vi "CS_cRIO-PB_MSAC2_DPV1-InitiateReq.vi"(0 "FPGA VI Reference":T6, 5 "Slave":i8, 7 "Initiate data":T7={"Communication ref.:"=0, "Send timeout (x10ms):"=0, "Feat. supp. 1:"=0, "Feat. supp. 2:"=0, "Profile feat. supp. 1:"=0, "Profile feat. supp. 2:"=0, "Profile ID number:"=0, "Addional address parameter"={"S-Type"=FALSE, "S-Length:"=2, "D-Type"=FALSE, "D-Length:"=2, "Data:"=[0, 0, 0, 0]}} {"Addional address parameter"."D-Length:" format="%0.0f"; "Addional address parameter"."S-Length:" format="%0.0f"; "Addional address parameter"."Data:" format="%.0x"; "Feat. supp. 2:" format="%.0x"; "Feat. supp. 1:" format="%.0x"; "Profile feat. supp. 2:" format="%.0x"; "Profile feat. supp. 1:" format="%.0x"; "Profile ID number:" format="%.0x"; "Send timeout (x10ms):" format="%0.0f"; "Communication ref.:" min=1 max=49 format="%0.0f"}, 11 "Error":errorcluster) -> (4 "FPGA VI Reference out":T6, 6 "Result":T1, 8 "Initiate response data":T2 {"Error data"."Error decode:" format="%.0x"; "Error data"."Remote address:" format="%0.0f"; "Error data"."Communication ref.:" format="%0.0f"; "Abort data"."Reasoncode:" format="%.0x"; "Abort data"."Instance:" format="%.0x"; "Abort data"."Additional detail:" format="%04x"; "Abort data"."Subnet:" format="%.0x"; "Abort data"."Response SAP:" format="%0.0f"; "Abort data"."Remote address:" format="%0.0f"; "Initiate data"."Addional address parameter"."D-Length:" format="%0.0f"; "Initiate data"."Addional address parameter"."S-Length:" format="%0.0f"; "Initiate data"."Addional address parameter"."Data:" format="%.0x"; "Initiate data"."Feat. supp. 2:" format="%.0x"; "Initiate data"."Feat. supp. 1:" format="%.0x"; "Initiate data"."Profile feat. supp. 2:" format="%.0x"; "Initiate data"."Profile feat. supp. 1:" format="%.0x"; "Initiate data"."Profile ID number:" format="%.0x"; "Initiate data"."Remote add.:" format="%0.0f"; "Initiate data"."Communication ref.:" format="%0.0f"}, 15 "Error out":errorcluster)   [LabVIEW 2013, in "dynamic profibus.lvlib"]
doc: "Establishes a DPV1 connection with the DP Slave.\n\nFPGA VI Reference:\nReference of the FPGA VI.\n\nSlave:\nPROFIBUS address of the DPV1 Slave. \n\n\nInitiate data:\n\nCommunication ref.:\nThe communication reference (range 1...49) is a local identifier and must be used for reading or writing DPV1 data with this DPV1 Slave. Multiple communication references for one DPV1 Slave is not allowed.\n\nSend timeout:\nAssigns the connection time out in multiples of 10mS. After connection setup the DPV1 Master polls the DPV1 Slave to see if the connection is o.k. If the DPV1 Slave does not respond, the timer expires and the connection is aborted by the DPV1 Master.\n\nThe following parameters are additional DPV1 Slave and network parameters and are set to working default values which need only to be changed in special cases. Please refer to the DPV1 Slave documentation for details.\n\nFeat. supp. 1:\nFeat. supp. 2:\nProfile feat. supp. 1:\nProfile feat. supp. 2:\nProfile ID number:\n\nAdditional address parameter:\nS-Type:\nS-Length:\nD-Type:\nD-Length:\nData:\n\n\nFPGA VI Reference out:\nIs a copy of the FPGA VI Reference .\n\nResult:\nSuccess: The DPV1 Slave responded with a positive confirmation, connection is established.\nAbort: Connection is aborted by DPV1 Master or DPV1 Slave. Check Abort data.\nError: DPV1 Error occured. Check Error data.\n\n\nInitiate response data:\nThe following values are returned by the Initiate_Req function in case of a positive confirmation (DPV1 Slave accepts connection).\n\nCommunication ref.:\nThe selected communication reference.\n\nRemote add.:\nProfibus address of the DPV1 Slave.\n\nFeat. supp. 1:\nFeat. supp. 2:\nProfile feat. supp. 1:\nProfile feat. supp. 2:\nProfile ID number:\n\nAdditional address parameter:\nS-Type:\nS-Length:\nD-Type:\nD-Length:\nData:\n\nAdditional DPV1 Slave and network parameters returned\n\n\nAbort data:\n\nThe following values are returned by the Initiate_Req function in case of a negative confirmation (DPV1 Slave refuses connection or DPV1 Master refuses service)\n\nRemote address:\nProfibus address of the DPV1 Slave.\n\nResponse SAP:\nCommunication SAP of the DPV1 Slave.\n\nLocally generated:\nTRUE indicates, that the DPV1 Master refused the connection.\n\nSubnet: Always 0\nInstance: 0 = FDL; 1 = MSAC_C2; 2 = User\n\nReasoncode: \n\nFDL (Instance)\n1 = UE ; 2 = RR ; 3 = RS ; 9 = NR ; 10 = DH ; 11 = LR ; 12 = RDL ; 13 = RDH ; 14 = DS ; 15 = NA \nThe FDL error codes are described in the COMSOFT DP_DPV1_e.pdf document, chapter 5 or in the PROFIBUS standard, FDL Layer.\n\nMSAC_C2 (Instance)\n1 = ABT_SE sequence error; service not allowed in this state\n2 = ABT_FE invalid request PDU received\n3 = ABT_TO timeout of the connection\n4 = ABT_RE invalid response PDU received\n5 = ABT_IV invalid service from USER\n6 = ABT_STO Send_Timeout requested was to small\n7 = ABT_IA invalid additional address information\n8 = ABT_OC waiting for FDL_DATA_REPLY.con\n\nAdditional_Detail:\nThis parameter contains the Send_Timeout received in the RM-REQ-PDU if the instance is MSAC_C2 and the Reason_Code is ABT_STO\n\nUser (Instance)\nManufacturer specific\n\n\nError data:\n\nThe error tab displays DPV1 communication errors.\n\nCommunication ref.:\nThe selected communication reference.\n\nRemote address:\nProfibus address of the DPV1 Slave.\n\nError decode:\n0 to 127 = reserved ; 128 = DPV1 ; 129 to 253 = reserved ; 254 = PROFIBUS FMS ; 255 = HART®\n\nError code 1:\nBit 0 - 3 is the error code, Bit 4 - 7 is the error class\n\nBit 4-7 = 0-9: reserved\n\nBit 4-7 = 10 and Bit 0-3 = 0: read error; 1: write error; 2: module failure; 3 - 7: reserved; 8: version conflict ; 9: feature not supported ; 10 to 15: user specific\n\nBit 4-7 = 11 and Bit 0-3 = 0: invalid index; 1: write length error; 2: invalid slot; 3: type conflict; 4: invalid area; 5: state conflict; 6: access denied; 7: invalid range; 8: invalid parameter; 9: invalid type; 10 to 15: user specific;\n\nBit 4-7 = 12 and Bit 0-3 = 0: read constrain conflict; 1: write constrain conflict; 2: resource busy; 3: resource unavailable; 4 to 7 = reserved; 8 to 15: user specific;\n\nBit 4-7 = 13-15: user specific: \n\nError code 2:\nUser specific\n\n\nError:\nPreceeding error conditions. If an error has already occurred, the VI returns the value of the error in Error out.\n\nError out:\nError: TRUE if an error occurred.\nStatus: Error code\nInfo: Error description"
uses:
  dynamic profibus.lvlib
  CS_cRIO-PB_DP-Master_FPGA-Reference.ctl
  Examples/SubVIs/CS_PB_DPV1_InitiateResData.ctl
  Examples/SubVIs/CS_PB_DPV1_InitiateConData.ctl
  Examples/SubVIs/CS_PB_DPV1_AbortIndData.ctl
  Examples/SubVIs/CS_PB_DPV1_ErrorData.ctl
  Examples/SubVIs/CS_PB_DPV1_Result.ctl
  Examples/SubVIs/CS_PB_DPV1_InitiateReqData.ctl
panel:
  # "- Enter a value of 1000 for the parameter Send timeout. Send timeout sets the internal timers for the connection monitoring and the response timeout. The Send timeout value is assigned in multiples of 10 mS, 1000 means 10000 mS or 10 s.\n\n- Leave all other parameters unchanged.\n\n- Click the DPV1 Initiate button. After the service is completed, the Result has to display Success, what means that the DPV1 connection was successfully established to the DP Slave.\n\nIf the Result does not display Success, check the Abort and Error section. See Context Help for detailed description of error checking."
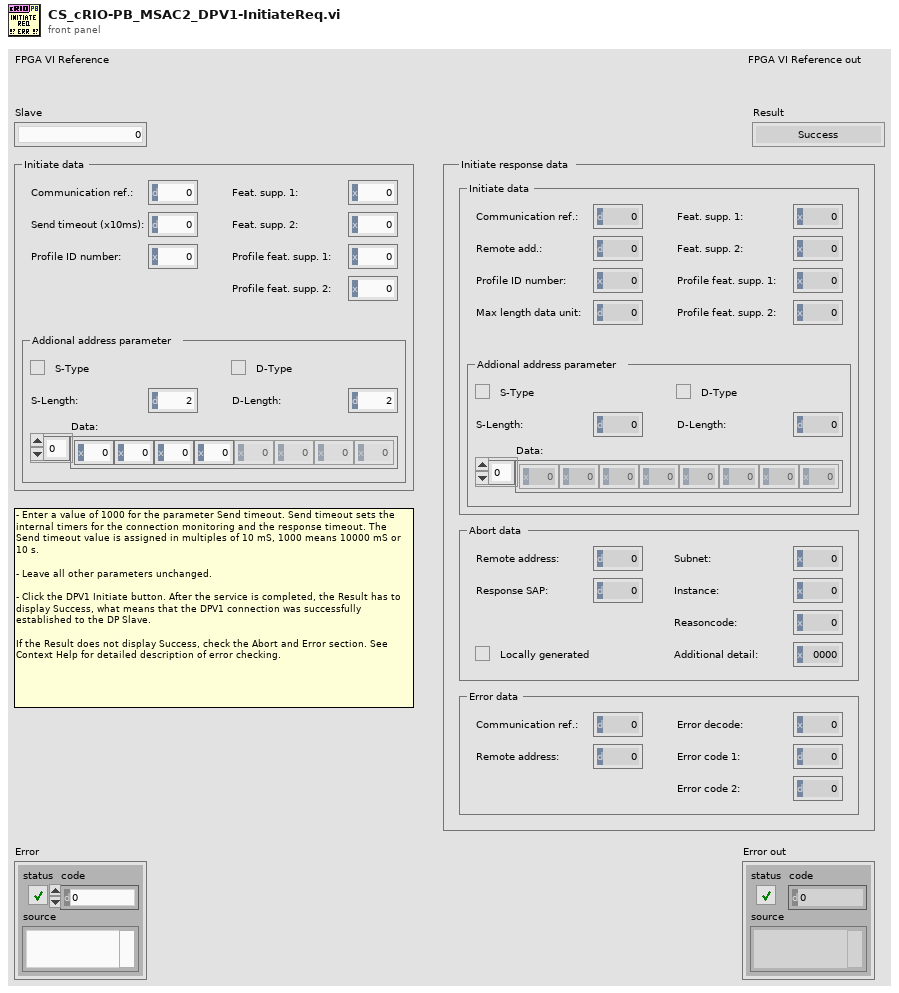
[diagram p1: front panel]
types:
  T1 = typedef "CS_PB_DPV1_Result.ctl" = enum16{"Success", "Abort", "Error"}
  T2 = typedef "CS_PB_DPV1_InitiateResData.ctl" = cluster{"Initiate data":T3, "Abort data":T4, "Error data":T5}
  T3 = typedef "CS_PB_DPV1_InitiateConData.ctl" = cluster{"Communication ref.:":u8, "Remote add.:":u8, "Feat. supp. 1:":u8, "Feat. supp. 2:":u8, "Profile feat. supp. 1:":u8, "Profile feat. supp. 2:":u8, "Profile ID number:":u16, "Addional address parameter":cluster{"S-Type":bool, "S-Length:":u8, "D-Type":bool, "D-Length:":u8, "Data:":u8[]}, "Max length data unit:":u8}
  T4 = typedef "CS_PB_DPV1_AbortIndData.ctl" = cluster{"Remote address:":u8, "Response SAP:":u8, "Locally generated":bool, "Subnet:":u8, "Instance:":u8, "Reasoncode:":u8, "Additional detail:":u16}
  T5 = typedef "CS_PB_DPV1_ErrorData.ctl" = cluster{"Communication ref.:":u8, "Remote address:":u8, "Error decode:":u8, "Error code 1:":u8, "Error code 2:":u8}
  T6 = typedef "dynamic profibus.lvlib/CS_cRIO-PB_DP-Master_FPGA-Reference.ctl" = refnum<k20>
  T7 = typedef "CS_PB_DPV1_InitiateReqData.ctl" = cluster{"Communication ref.:":u8, "Send timeout (x10ms):":u16, "Feat. supp. 1:":u8, "Feat. supp. 2:":u8, "Profile feat. supp. 1:":u8, "Profile feat. supp. 2:":u8, "Profile ID number:":u16, "Addional address parameter":cluster{"S-Type":bool, "S-Length:":u8, "D-Type":bool, "D-Length:":u8, "Data:":u8[]}}
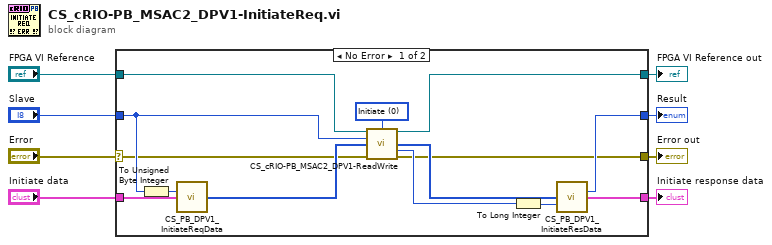
[diagram p0: block diagram]
diagram:
  n1 = case shown="No Error" "Error" {
    selector: "Error" -> [w19 w23]
    tunnel: "Slave" -> [w22 _]
    tunnel: "FPGA VI Reference" -> [w17 w24]
    tunnel: [w18 w24] -> w4
    tunnel: [w9 w23] -> w2
    tunnel: [w11 _] -> w1
    tunnel: [w10 _] -> w3
    tunnel: "Initiate data" -> [w14 _]
    frame No Error {
      w16 = i8 0 items=["Initiate", "Read", "Write", "Abort"] ("DPV1-Service")
      n2 = To Unsigned Byte Integer(number=w22) -> (unsigned 8bit integer=w15:u8)
      n3 = call "CS_PB_DPV1_InitiateReqData.vi"("Profibus address:"=w15, "Initiate data"=w14) -> ("Request data"=w21:u8[])  [unwired: 13 in]
      n4 = call "CS_cRIO-PB_MSAC2_DPV1-ReadWrite.vi"("FPGA VI Reference"=w17, "DPV1-Service"=w16, "Slave"=w22, "Data"=w21, "Error"=w19) -> ("FPGA VI Reference out"=w18:T6, "Data out"=w12:u8[], "Status"=w20:u8, "Error out"=w9:errorcluster)  [unwired: 7 in]
      n5 = To Long Integer(number=w20) -> (32bit integer=w13:i32)
      n6 = call "CS_PB_DPV1_InitiateResData.vi"("Response data"=w12, "Status"=w13) -> ("Result"=w10:T1, "Initiate response data"=w11:T2)  [unwired: 12 in]
    }
    frame Error {
    }
  }
  "Error out" <- w2
  "FPGA VI Reference out" <- w4
  "Initiate response data" <- w1
  "Result" <- w3
